vi "GUNSC_LibAddAmp_bak.vi"(1 "correctedxstart":i32, 2 "correctedystart":i32, 5 "Amplifier":T1={"number"=0, "type"=0, "rotated"=0, "fliped"=0, "FPAcoord"={"xstart"=1, "ystart"=1}, "Physical_size"={"columns"=0, "rows"=0}, "predata"={"columns"=0, "rows"=0}, "postdata"={"columns"=0, "rows"=0}, "Req ROIs"=[], "Corr ROI"=[], "Detnumber"=0, "ampID"="", "discard"=0} {"fliped" items=["none", "horizontal", "vertical"]; "type" items=["LL", "LR", "UL", "UR"]}, 7 "extension":i32, 11 "error in (no error)":errorcluster) -> (6 "return value":i32, 15 "error out":errorcluster)   [LabVIEW 2014]
uses:
  GEOM/private/vis/GEOM_Amplifier.ctl
  GEOM/private/vis/GEOM_AmpType.ctl
  GEOM/private/vis/GEOM_ROI.ctl
  GEOM/private/vis/GEOM_Coords.ctl
  public/c/lib/libunsc.so
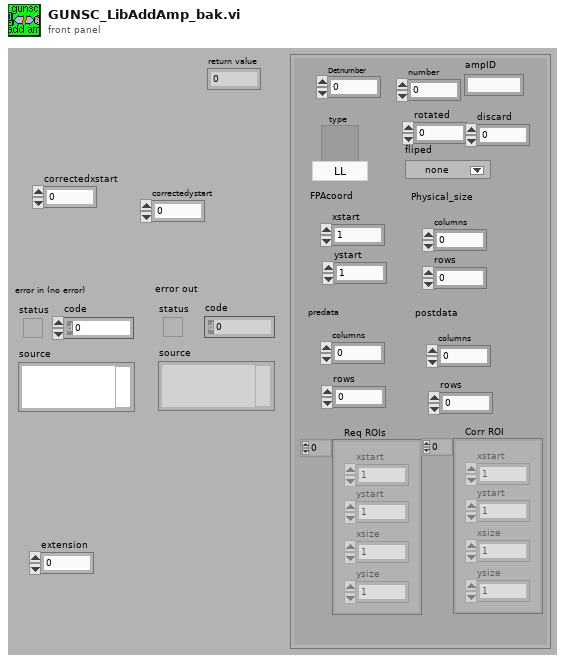
[diagram p1: front panel]
types:
  T1 = typedef "GEOM_Amplifier.ctl" = cluster{"number":i32, "type":T2, "rotated":i16, "fliped":u16, "FPAcoord":cluster{"xstart":i32, "ystart":i32}, "Physical_size":cluster{"columns":i32, "rows":i32}, "predata":cluster{"columns":i32, "rows":i32}, "postdata":cluster{"columns":i32, "rows":i32}, "Req ROIs":T3, "Corr ROI":T3, "Detnumber":i32, "ampID":string, "discard":i32}
  T2 = typedef "GEOM_AmpType.ctl" = u16
  T3 = typedef "GEOM_ROI.ctl" = T4[]
  T4 = typedef "GEOM_Coords.ctl" = cluster{"xstart":u32, "ystart":u32, "xsize":u32, "ysize":u32}
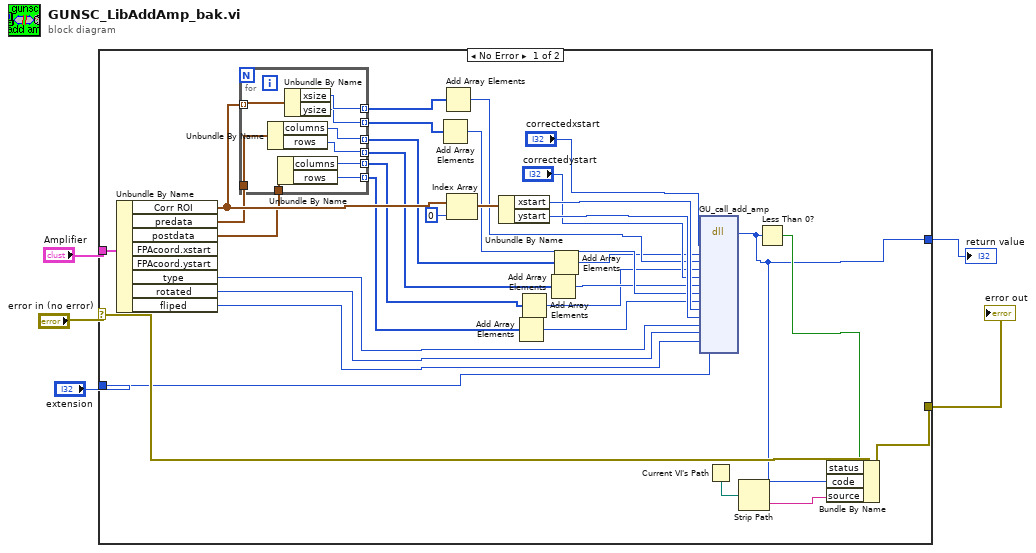
[diagram p0: block diagram]
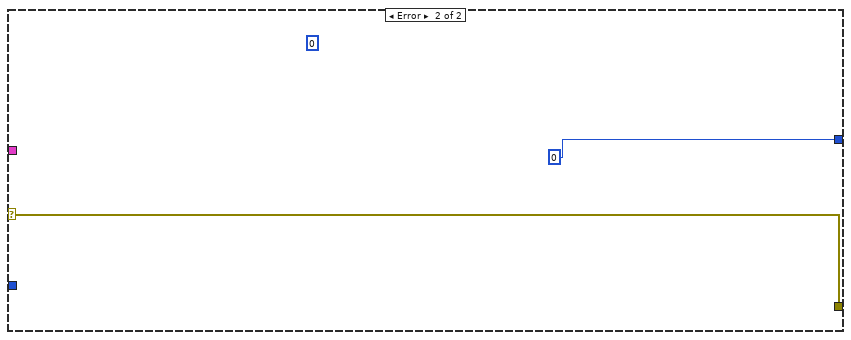
[diagram p2: hidden frame]
diagram:
  n1 = case shown="No Error" "error in (no error)" {
    selector: "error in (no error)" -> [w37 w48]
    tunnel: [w28 0] -> w5
    tunnel: [w34 w48] -> w3
    tunnel: "Amplifier" -> [w33 _]
    tunnel: "extension" -> [w27 _]
    frame No Error {
      n2 = Unbundle By Name(w33) -> ("Corr ROI"=w20:T3, "predata"=w13:cluster{"columns":i32, "rows":i32}, "postdata"=w12:cluster{"columns":i32, "rows":i32}, "type"=w31:T2, "rotated"=w30:i16, "fliped"=w29:u16)  [unwired: 2 out]
      n3 = for {
        tunnel: w20 -> [w46] mode=indexing
        tunnel: [w45] -> w19 mode=indexing
        tunnel: [w44] -> w18 mode=indexing
        tunnel: w13 -> [w43]
        tunnel: w12 -> [w42]
        tunnel: [w41] -> w11 mode=indexing
        tunnel: [w40] -> w10 mode=indexing
        tunnel: [w39] -> w9 mode=indexing
        tunnel: [w38] -> w6 mode=indexing
        n4 = Unbundle By Name(w43) -> ("columns"=w41:i32, "rows"=w40:i32)
        n5 = Unbundle By Name(w42) -> ("columns"=w39:i32, "rows"=w38:i32)
        n6 = Unbundle By Name(w46) -> ("xsize"=w45:u32, "ysize"=w44:u32)
      }
      n7 = Add Array Elements(numeric array=w18) -> (sum=w16:u32)
      n8 = Add Array Elements(numeric array=w19) -> (sum=w17:u32)
      n9 = Index Array(array=w20, index=0) -> (element=w25:T4)
      n10 = Unbundle By Name(w25) -> ("xstart"=w24:u32, "ystart"=w23:u32)
      n11 = Add Array Elements(numeric array=w6) -> (sum=w7:i32)
      n12 = Add Array Elements(numeric array=w9) -> (sum=w8:i32)
      n13 = Add Array Elements(numeric array=w10) -> (sum=w14:i32)
      n14 = Add Array Elements(numeric array=w11) -> (sum=w15:i32)
      n15 = dll-call lib="home/sispi/Panview-1.13.0-64b/PAN/Modules/GUNSC/public/c/lib/libunsc.so" fn="GU_call_add_amp"("xstart"="correctedxstart", "precols"=w15, "datacols"=w17, "postcols"=w8, "ystart"="correctedystart", "prerows"=w14, "datarows"=w16, "postrows"=w7, "xdetstart"=w24, "ydetstart"=w23, "type"=w31, "rotate"=w30, "flip"=w29, "extension"=w27) -> ("return type"=w28:i32)  [unwired: 16 in, 3 out]
      n16 = Current VI's Path() -> (path=w36:path)
      n17 = Strip Path(path=w36) -> (name=w35:string)  [unwired: 1 out]
      n18 = Less Than 0?(x=w28) -> (x < 0?=w32:bool)
      n19 = Bundle By Name(cluster=w37, "status"=w32, "code"=w28, "source"=w35) -> (w34:errorcluster)
    }
    frame Error {
      (unwired) 0
    }
  }
  "return value" <- w5
  "error out" <- w3
